vi "SeCrTs-RT_DAQ_- Copy.vi"(8 "error in":errorcluster, 9 "er":refnum<queue>, 11 "Data FIFO Ref":T1) -> (0 "error out":errorcluster)   [LabVIEW 2022 SP3]
uses:
  RT Controls/SeCrTs-Data FIFO.ctl
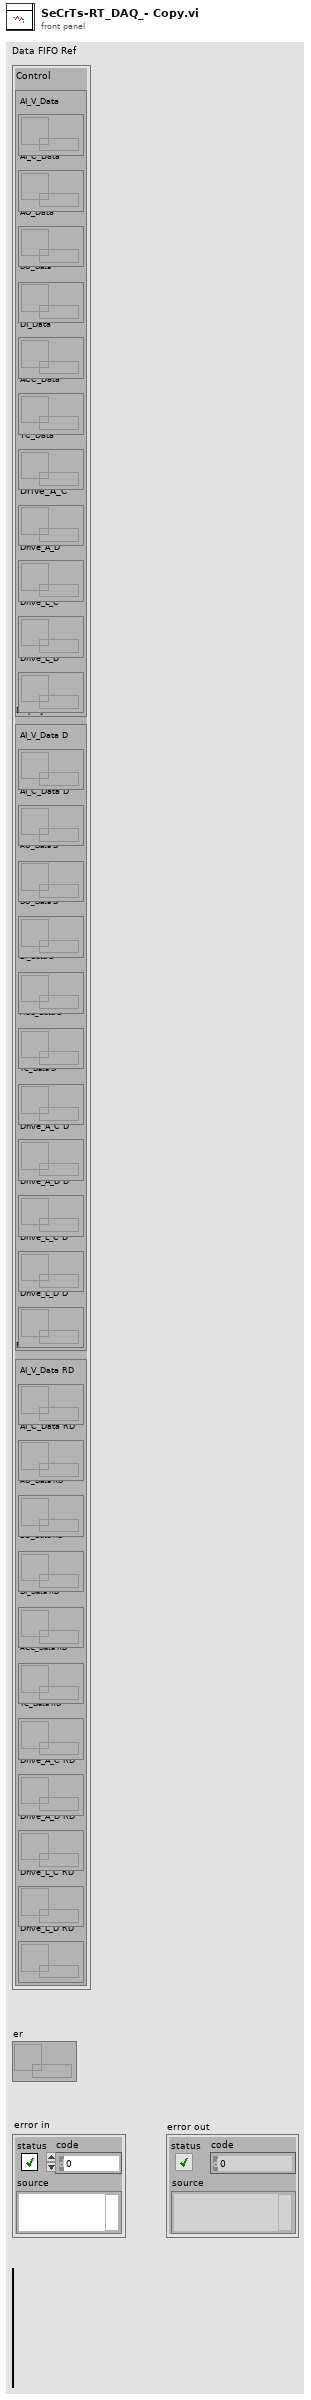
[diagram p1: front panel]
types:
  T1 = typedef "SeCrTs-Data FIFO.ctl" = cluster{"Control":cluster{"AI_V_Data":refnum<queue>, "AI_C_Data":refnum<queue>, "AO_Data":refnum<queue>, "DO_Data":refnum<queue>, "DI_Data":refnum<queue>, "ACC_Data":refnum<queue>, "TC_Data":refnum<queue>, "Drive_A_C":refnum<queue>, "Drive_A_D":refnum<queue>, "Drive_L_C":refnum<queue>, "Drive_L_D":refnum<queue>}, "Display":cluster{"AI_V_Data D":refnum<queue>, "AI_C_Data D":refnum<queue>, "AO_Data D":refnum<queue>, "DO_Data D":refnum<queue>, "DI_Data D":refnum<queue>, "ACC_Data D":refnum<queue>, "TC_Data D":refnum<queue>, "Drive_A_C D":refnum<queue>, "Drive_A_D D":refnum<queue>, "Drive_L_C D":refnum<queue>, "Drive_L_D D":refnum<queue>}, "RD":cluster{"AI_V_Data RD":refnum<queue>, "AI_C_Data RD":refnum<queue>, "AO_Data RD":refnum<queue>, "DO_Data RD":refnum<queue>, "DI_Data RD":refnum<queue>, "ACC_Data RD":refnum<queue>, "TC_Data RD":refnum<queue>, "Drive_A_C RD":refnum<queue>, "Drive_A_D RD":refnum<queue>, "Drive_L_C RD":refnum<queue>, "Drive_L_D RD":refnum<queue>}}
  T2 = cluster{"AO config":cluster{"Channel_Name":string, "Channel_Number":string, "Default_Value":dbl, "Units":string}[], "AI config":cluster{"Channel_Name":string, "Channel_Number":string, "Pre_Scale_min":dbl, "Pre_Scale_max":dbl, "Sensor_min":dbl, "Sensor_max":dbl, "Units":string}[], "DI config":cluster{"Channel_Name":string, "Channel_Number":string, "Default_Value":bool, "DI invert?":bool}[], "DO config":cluster{"Channel_Name":string, "Channel_Number":string, "Default_Value":bool, "DO invert?":bool}[], "TC config":cluster{"Channel_Name":string, "Channel_Number":string, "Pre_Scale_min":dbl, "Pre_Scale_max":dbl, "units":i32, " type":i32}[], "ACC config":cluster{"Channel_Name":string, "Channel_Number":string, "Pre_Scale_min":dbl, "Pre_Scale_max":dbl, "Terminal configuration":i32, "Sensitivity":dbl, "Sensitivity units":i32}[], "SG config":cluster{"Channel_Name":string, "Channel_Number":string, "Pre_Scale_min":dbl, "Pre_Scale_max":dbl}[], "Strain Gauge Settings":cluster{"poisson ratio":dbl, "nominal gage resistance":dbl, "gage factor":dbl}, "Bridge Settings":cluster{"voltage excitation value":dbl, "voltage excitation source":i32, "initial bridge voltage":dbl, "lead wire resistance":dbl, "strain configuration":i32}, "Sample Rate":cluster{"AI Sample Rate":dbl[], "AO Sample Rate":dbl[], "DI Sample Rate":dbl[], "TC Sample Rate":dbl[], "DO Sample Rate":dbl[], "SG Sample Rate":dbl[], "ACC Sample Rate":dbl[]}}
  T3 = enum16{"Initialize", "Create Task", "Start", "Acquire", "Stop", "Exit"}
  T4 = cluster{"AI_Task":refnum<k21>, "AO_Task":refnum<k21>, "DI_Task":refnum<k21>, "DO_Task":refnum<k21>, "ACC_Task":refnum<k21>, "TC_Task":refnum<k21>, "AI_V_Task":refnum<k21>}
  T5 = cluster{"Start DAQ":bool, "Stop DAQ":bool, "RT Stop":bool, "RT Exit":bool, "Start Seq":bool}
  T6 = cluster{"AO config":cluster{"Channel_Name":string, "Channel_Number":string, "Default_Value":dbl, "Units":string}[], "AI config":cluster{"Channel_Name":string, "Channel_Number":string, "Pre_Scale_min":dbl, "Pre_Scale_max":dbl, "Sensor_min":dbl, "Sensor_max":dbl, "Units":string}[], "DI config":cluster{"Channel_Name":string, "Channel_Number":string, "Default_Value":bool, "DI invert?":bool}[], "DO config":cluster{"Channel_Name":string, "Channel_Number":string, "Default_Value":bool, "DO invert?":bool}[], "TC config":cluster{"Channel_Name":string, "Channel_Number":string, "Pre_Scale_min":dbl, "Pre_Scale_max":dbl, "units":i32, "thermocouple type":i32}[], "ACC config":cluster{"Channel_Name":string, "Channel_Number":string, "Pre_Scale_min":dbl, "Pre_Scale_max":dbl, "Terminal configuration":i32, "Sensitivity":dbl, "Sensitivity units":i32}[], "SG config":cluster{"Channel_Name":string, "Channel_Number":string, "Pre_Scale_min":dbl, "Pre_Scale_max":dbl}[], "Strain Gauge Settings":cluster{"poisson ratio":dbl, "nominal gage resistance":dbl, "gage factor":dbl}, "Bridge Settings":cluster{"voltage excitation value":dbl, "voltage excitation source":i32, "initial bridge voltage":dbl, "lead wire resistance":dbl, "strain configuration":i32}, "Sample Rate":cluster{"AI Sample Rate":dbl[], "AO Sample Rate":dbl[], "DI Sample Rate":dbl[], "TC Sample Rate":dbl[], "DO Sample Rate":dbl[], "SG Sample Rate":dbl[], "ACC Sample Rate":dbl[]}}
  T7 = cluster{"Channel_Name":string, "Channel_Number":string, "Pre_Scale_min":dbl, "Pre_Scale_max":dbl, "Sensor_min":dbl, "Sensor_max":dbl, "Units":string}[]
  T8 = cluster{"Channel_Name":string, "Channel_Number":string, "Default_Value":dbl, "Units":string}[]
  T9 = cluster{"Channel_Name":string, "Channel_Number":string, "Default_Value":bool, "DI invert?":bool}[]
  T10 = cluster{"Channel_Name":string, "Channel_Number":string, "Default_Value":bool, "DO invert?":bool}[]
  T11 = cluster{"Channel_Name":string, "Channel_Number":string, "Pre_Scale_min":dbl, "Pre_Scale_max":dbl, "Terminal configuration":i32, "Sensitivity":dbl, "Sensitivity units":i32}[]
  T12 = cluster{"Channel_Name":string, "Channel_Number":string, "Pre_Scale_min":dbl, "Pre_Scale_max":dbl, "units":i32, " type":i32}[]
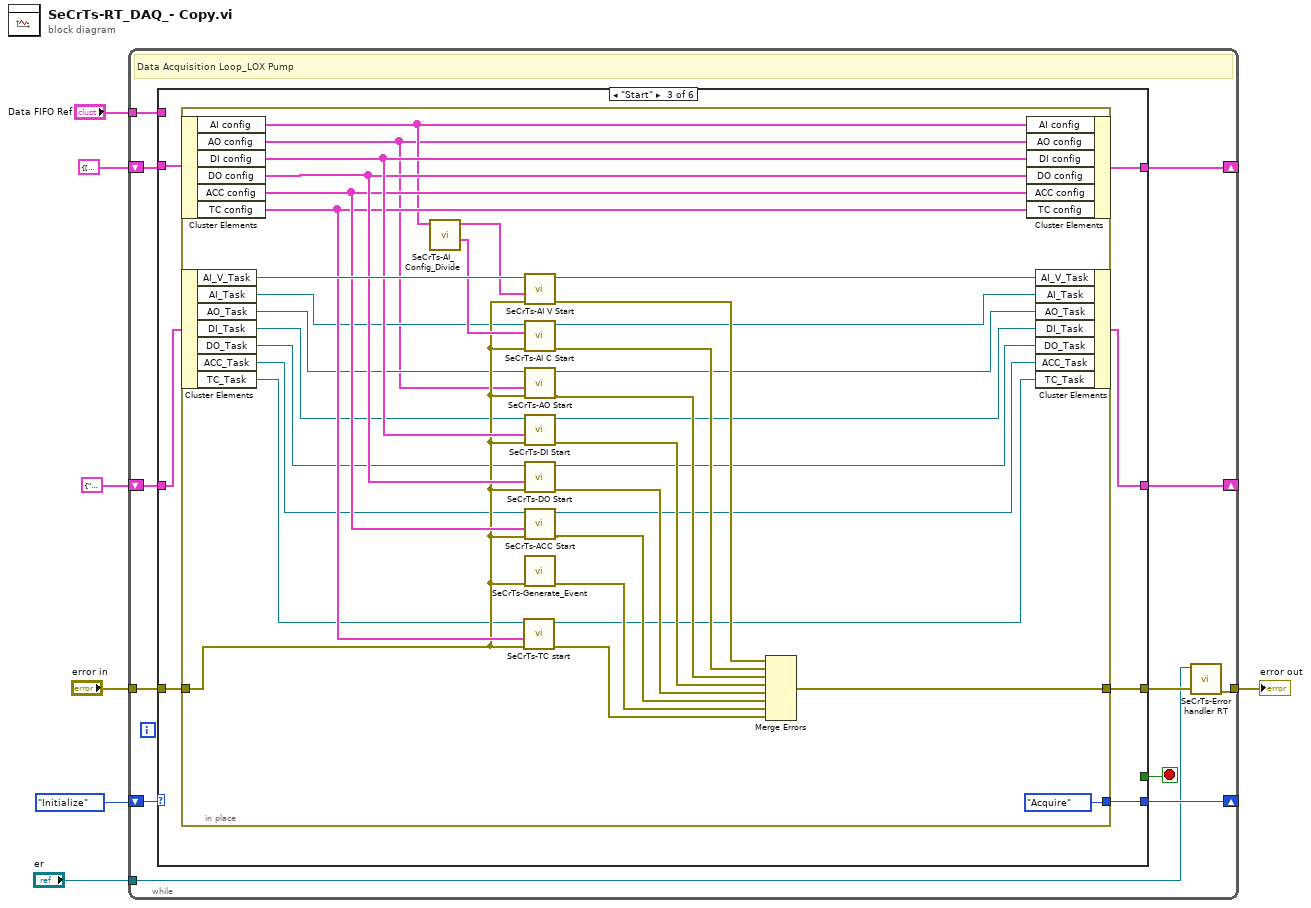
[diagram p0: block diagram]
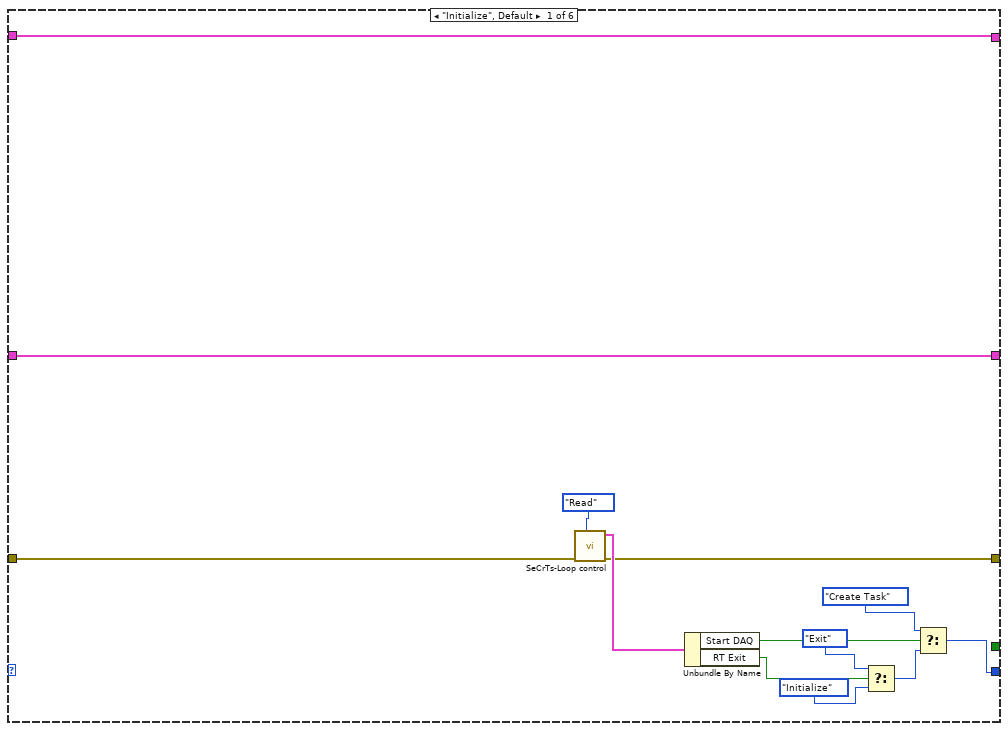
[diagram p2: hidden frame]
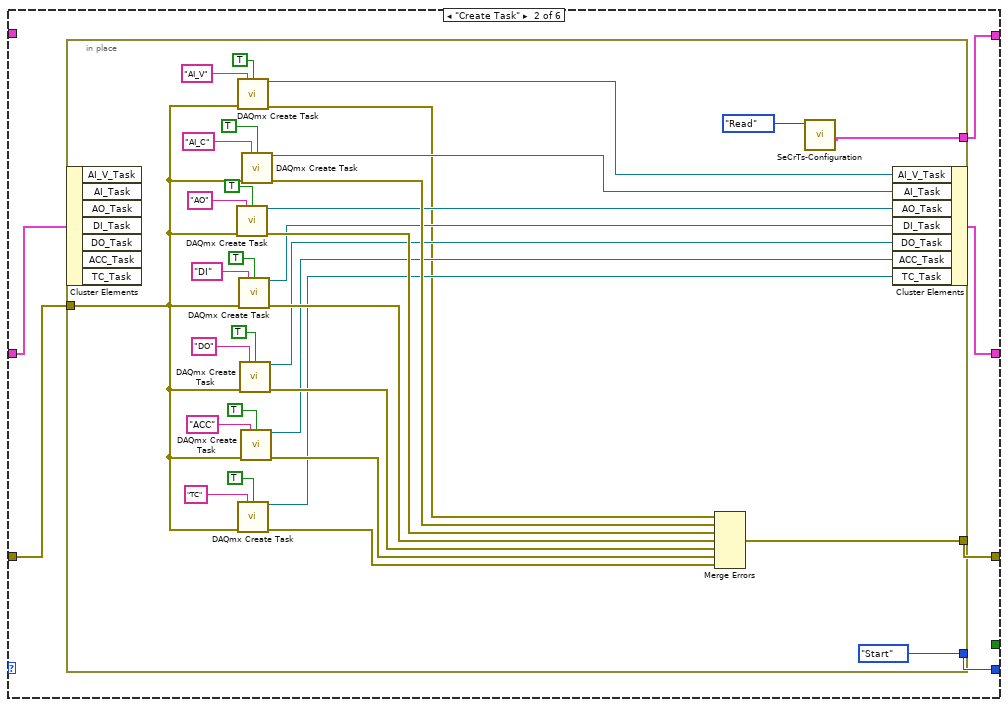
[diagram p3: hidden frame]
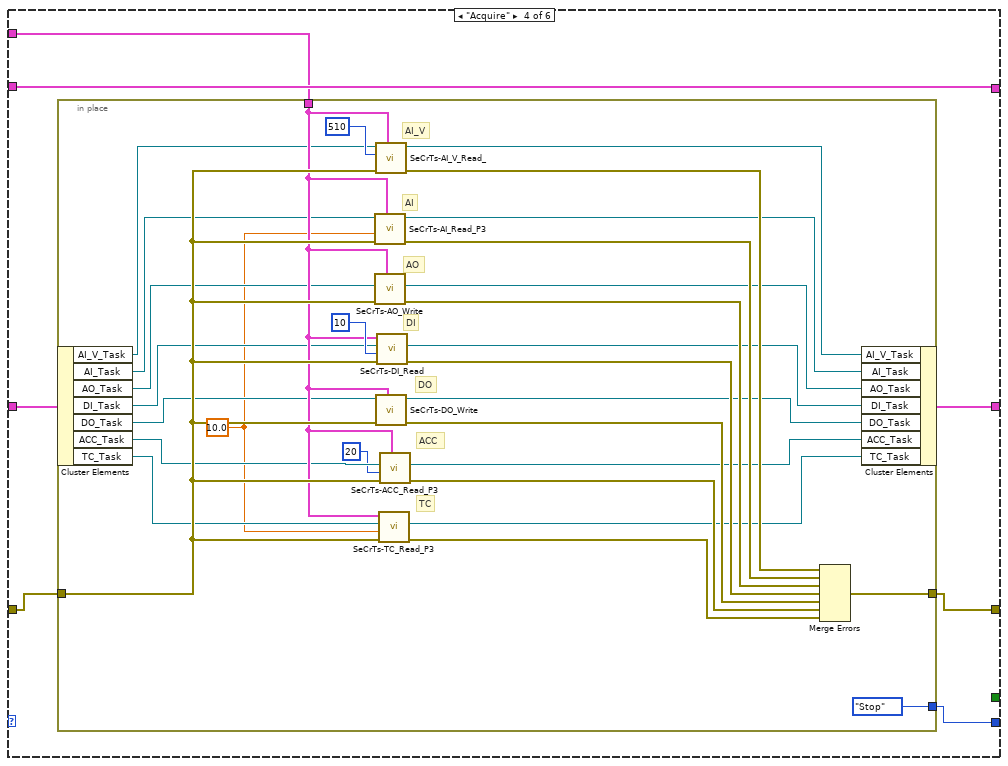
[diagram p4: hidden frame]
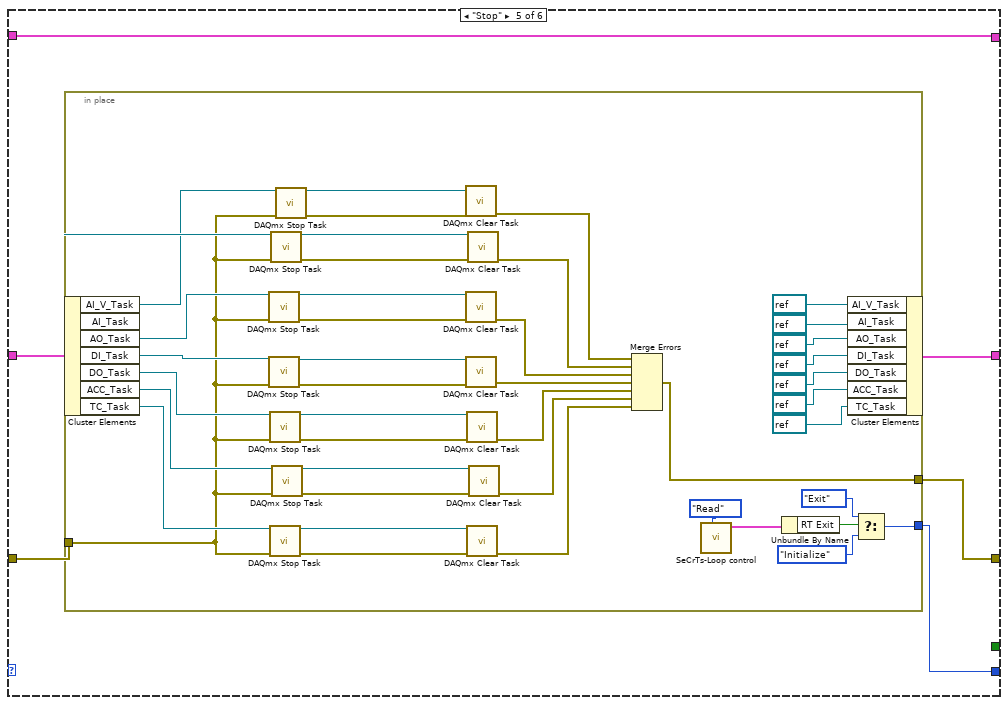
[diagram p5: hidden frame]
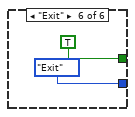
[diagram p6: hidden frame]
diagram:
  n1 = while {
    shift-right: [w17] -> _
    shift-left: T3."Initialize" -> [w19]
    tunnel: "error in" -> [w18]
    tunnel: [w8] -> w6
    shift-right: [w14] -> _
    shift-left: T2 {"AO config"=[], "AI config"=[], "DI config"=[], "DO config"=[], "TC config"=[], "ACC config"=[], "SG config"=[], "Strain Gauge Settings"={"poisson ratio"=0.0, "nominal gage resistance"=0.0, "gage factor"=0.0}, "Bridge Settings"={"voltage excitation value"=0.0, "voltage excitation source"=0, "initial bridge voltage"=0.0, "lead wire resistance"=0.0, "strain configuration"=0}, "Sample Rate"={"AI Sample Rate"=[], "AO Sample Rate"=[], "DI Sample Rate"=[], "TC Sample Rate"=[], "DO Sample Rate"=[], "SG Sample Rate"=[], "ACC Sample Rate"=[]}} ("Config out") -> [w15]
    shift-right: [w12] -> _
    shift-left: T4 {"AI_Task"="", "AO_Task"="", "DI_Task"="", "DO_Task"="", "ACC_Task"="", "TC_Task"="", "AI_V_Task"=""} -> [w16]
    tunnel: "Data FIFO Ref" -> [w11]
    tunnel: "er" -> [w9]
    stop <- w13 stop-if-true
    # "Data Acquisition Loop_LOX Pump"
    n2 = case shown="\"Start\"" w19 {
      tunnel: w18 -> [w21 w37 w77 w117 w151 _]
      tunnel: [w20 w36 w73 w116 w152 _] -> w10
      tunnel: [w31 w35 w78 w118 w153 T3."Exit"] -> w17
      tunnel: w16 -> [w23 w34 w76 w113 w150 _]
      tunnel: w15 -> [w22 _ w75 w115 w148 _]
      tunnel: [w22 w38 w74 w115 w148 _] -> w14
      tunnel: [_ _ _ _ _ TRUE] -> w13
      tunnel: [w23 w33 w72 w112 w149 _] -> w12
      tunnel: w11 -> [_ _ _ w114 _ _]
      frame "Initialize", Default {
        n3 = call "SeCrTs-Loop control.vi"("Action"=enum16{"Init", "Write", "Read"}."Read", "error in (no error)"=w21) -> ("error Out"=w20:errorcluster, "Loop Control out"=w27:T5)  [unwired: 8 in]
        n4 = Unbundle By Name(w27) -> ("Start DAQ"=w26:bool, "RT Exit"=w25:bool)
        n5 = Select(t=T3."Exit", s=w25, f=T3."Initialize") -> (s? t:f=w28:T3)
        n6 = Select(t=T3."Create Task", s=w26, f=w28) -> (s? t:f=w31:T3)
      }
      frame "Create Task" {
        n7 = in-place "In Place Element Structure" {
          in-place-border: [w50] -> w38
          in-place-border: w37 -> [w39]
          in-place-border: [w60] -> w36
          in-place-border: [T3."Start"] -> w35
          n8 = in-place-cluster #1(w34) -> ()  [unwired: 7 out]
          n9 = call <vilib>:"DAQmx Create Task.vi"("new task name"="AO", "auto cleanup"=TRUE, "error in"=w39) -> ("task out"=w58:refnum<k21>, "error out"=w65:errorcluster)  [unwired: 11 in]
          n10 = call <vilib>:"DAQmx Create Task.vi"("new task name"="AI_V", "auto cleanup"=TRUE, "error in"=w39) -> ("task out"=w51:refnum<k21>, "error out"=w40:errorcluster)  [unwired: 11 in]
          n11 = call <vilib>:"DAQmx Create Task.vi"("new task name"="TC", "auto cleanup"=TRUE, "error in"=w39) -> ("task out"=w54:refnum<k21>, "error out"=w61:errorcluster)  [unwired: 11 in]
          n12 = call <vilib>:"DAQmx Create Task.vi"("new task name"="DI", "auto cleanup"=TRUE, "error in"=w39) -> ("task out"=w57:refnum<k21>, "error out"=w64:errorcluster)  [unwired: 11 in]
          n13 = call <vilib>:"DAQmx Create Task.vi"("new task name"="DO", "auto cleanup"=TRUE, "error in"=w39) -> ("task out"=w56:refnum<k21>, "error out"=w63:errorcluster)  [unwired: 11 in]
          n14 = call <vilib>:"DAQmx Create Task.vi"("new task name"="ACC", "auto cleanup"=TRUE, "error in"=w39) -> ("task out"=w55:refnum<k21>, "error out"=w62:errorcluster)  [unwired: 11 in]
          n15 = call <vilib>:"DAQmx Create Task.vi"("new task name"="AI_C", "auto cleanup"=TRUE, "error in"=w39) -> ("task out"=w59:refnum<k21>, "error out"=w71:errorcluster)  [unwired: 11 in]
          n16 = Merge Errors(w40, w71, w65, w64, w63, w62, w61) -> (w60:errorcluster)
          n17 = call "SeCrTs-Configuration.vi"("Enum"=enum16{"Write", "Read"}."Read") -> ("Config out"=w50:T6)  [unwired: 10 in]
          n18 = in-place-cluster #1("AI_V_Task"=w51, "AI_Task"=w59, "AO_Task"=w58, "DI_Task"=w57, "DO_Task"=w56, "ACC_Task"=w55, "TC_Task"=w54) -> (w33:T4)
        }
      }
      frame "Start" {
        n19 = in-place "In Place Element Structure" {
          in-place-border: [T3."Acquire"] -> w78
          in-place-border: w77 -> [w97]
          in-place-border: [w92] -> w73
          n20 = in-place-cluster #2(w75) -> ("AI config"=w104:T7, "AO config"=w79:T8, "DI config"=w108:T9, "DO config"=w107:T10, "ACC config"=w106:T11, "TC config"=w105:T12)
          n21 = in-place-cluster #3(w76) -> ("AI_V_Task"=w110:refnum<k21>, "AI_Task"=w91:refnum<k21>, "AO_Task"=w90:refnum<k21>, "DI_Task"=w89:refnum<k21>, "DO_Task"=w88:refnum<k21>, "ACC_Task"=w87:refnum<k21>, "TC_Task"=w86:refnum<k21>)
          n22 = call "SeCrTs-AI_Config_Divide.vi"("AI config"=w104) -> ("AI C"=w102:T7, "AI V"=w103:T7)  [unwired: 9 in]
          n23 = call "SeCrTs-TC start .vi"("error in"=w97, "TC config"=w105, "Refnum in"=w86) -> ("error out"=w93:errorcluster, "Refnum out"=w80:refnum<k21>)  [unwired: 7 in]
          n24 = call "SeCrTs-AI V Start .vi"("error in"=w97, "AI V"=w103, "Refnum in"=w110) -> ("error out"=w101:errorcluster, "Refnum out"=w109:refnum<k21>)  [unwired: 7 in]
          n25 = call "SeCrTs-AI C Start .vi"("error in"=w97, "AI C"=w102, "Refnum in"=w91) -> ("error out"=w100:errorcluster, "Refnum out"=w85:refnum<k21>)  [unwired: 7 in]
          n26 = call "SeCrTs-AO Start .vi"("error in"=w97, "AO config"=w79, "Refnum in"=w90) -> ("error out"=w99:errorcluster, "Refnum out"=w84:refnum<k21>)  [unwired: 7 in]
          n27 = call "SeCrTs-DI Start.vi"("error in"=w97, "DI config"=w108, "Refnum in"=w89) -> ("error out"=w98:errorcluster, "Refnum out"=w83:refnum<k21>)  [unwired: 7 in]
          n28 = call "SeCrTs-DO Start.vi"("error in"=w97, "DO config"=w107, "Refnum in"=w88) -> ("error out"=w96:errorcluster, "Refnum out"=w82:refnum<k21>)  [unwired: 7 in]
          n29 = call "SeCrTs-ACC Start.vi"("error in"=w97, "ACC config"=w106, "Refnum in"=w87) -> ("error out"=w95:errorcluster, "Refnum out"=w81:refnum<k21>)  [unwired: 7 in]
          n30 = call "SeCrTs-Generate_Event.vi"("error in"=w97) -> ("error out"=w94:errorcluster)  [unwired: 10 in]
          n31 = Merge Errors(w101, w100, w99, w98, w96, w95, w94, w93) -> (w92:errorcluster)
          n32 = in-place-cluster #2("AI config"=w104, "AO config"=w79, "DI config"=w108, "DO config"=w107, "ACC config"=w106, "TC config"=w105) -> (w74:T2)
          n33 = in-place-cluster #3("AI_V_Task"=w109, "AI_Task"=w85, "AO_Task"=w84, "DI_Task"=w83, "DO_Task"=w82, "ACC_Task"=w81, "TC_Task"=w80) -> (w72:T4)
        }
      }
      frame "Acquire" {
        n34 = in-place "In Place Element Structure" {
          in-place-border: [T3."Stop"] -> w118
          in-place-border: w117 -> [w138]
          in-place-border: [w146] -> w116
          in-place-border: w114 -> [w136]
          w120 = 10.0
          # "AO"
          # "ACC"
          # "AI_V"
          # "TC"
          # "DO"
          # "DI"
          # "AI"
          n35 = in-place-cluster #4(w113) -> ("AI_V_Task"=w121:refnum<k21>, "AI_Task"=w135:refnum<k21>, "AO_Task"=w134:refnum<k21>, "DI_Task"=w133:refnum<k21>, "DO_Task"=w132:refnum<k21>, "ACC_Task"=w131:refnum<k21>, "TC_Task"=w130:refnum<k21>)
          n36 = call "SeCrTs-AI_Read_P3.vi"("Data FIFO Ref"=w136, "error in (no error)"=w138, "Numeric"=w120, "AI_Task"=w135) -> ("error out"=w144:errorcluster, "task out"=w128:refnum<k21>)  [unwired: 4 in]
          n37 = call "SeCrTs-AO_Write.vi"("Data FIFO Ref"=w136, "error in (no error)"=w138, "AO_Task"=w134) -> ("error out"=w143:errorcluster, "task out"=w127:refnum<k21>)  [unwired: 7 in]
          n38 = call "SeCrTs-AI_V_Read_.vi"("Data FIFO Ref"=w136, "error in"=w138, "number of samples per channel"=510, "AI_V_Task"=w121) -> ("error out"=w145:errorcluster, "AI_V_Task"=w129:refnum<k21>)  [unwired: 6 in]
          n39 = call "SeCrTs-DO_Write.vi"("Data FIFO Ref"=w136, "error in (no error)"=w138, "Refnum in"=w132) -> ("error out"=w141:errorcluster, "Refnum out"=w125:refnum<k21>)  [unwired: 7 in]
          n40 = call "SeCrTs-DI_Read.vi"("error in (no error)"=w138, "number of samples per channel"=10, "DI_Task"=w133, "Data FIFO Ref"=w136) -> ("error out"=w142:errorcluster, "task out"=w126:refnum<k21>)  [unwired: 6 in]
          n41 = call "SeCrTs-TC_Read_P3.vi"("error in (no error)"=w138, "Numeric"=w120, "TC_Task"=w130, "Data FIFO Ref"=w136) -> ("error out"=w139:errorcluster, "task out"=w123:refnum<k21>)  [unwired: 6 in]
          n42 = call "SeCrTs-ACC_Read_P3.vi"("Data FIFO Ref"=w136, "error in (no error)"=w138, "number of samples per channel"=20, "ACC_Task"=w131) -> ("error out"=w140:errorcluster, "task out"=w124:refnum<k21>)  [unwired: 6 in]
          n43 = Merge Errors(w145, w144, w143, w142, w141, w140, w139) -> (w146:errorcluster)
          n44 = in-place-cluster #4("AI_V_Task"=w129, "AI_Task"=w128, "AO_Task"=w127, "DI_Task"=w126, "DO_Task"=w125, "ACC_Task"=w124, "TC_Task"=w123) -> (w112:T4)
        }
      }
      frame "Stop" {
        n45 = in-place "In Place Element Structure" {
          in-place-border: [w193] -> w153
          in-place-border: [w187] -> w152
          in-place-border: w151 -> [w168]
          n46 = in-place-cluster #5(w150) -> ("AI_V_Task"=w170:refnum<k21>, "AI_Task"=w179:refnum<k21>, "AO_Task"=w178:refnum<k21>, "DI_Task"=w181:refnum<k21>, "DO_Task"=w180:refnum<k21>, "ACC_Task"=w177:refnum<k21>, "TC_Task"=w176:refnum<k21>)
          n47 = call <vilib>:"DAQmx Stop Task.vi"("task/channels in"=w178, "error in"=w168) -> ("task out"=w175:refnum<k21>, "error out"=w192:errorcluster)  [unwired: 12 in]
          n48 = call <vilib>:"DAQmx Stop Task.vi"("task/channels in"=w181, "error in"=w168) -> ("task out"=w174:refnum<k21>, "error out"=w191:errorcluster)  [unwired: 12 in]
          n49 = call <vilib>:"DAQmx Stop Task.vi"("task/channels in"=w180, "error in"=w168) -> ("task out"=w173:refnum<k21>, "error out"=w190:errorcluster)  [unwired: 12 in]
          n50 = call <vilib>:"DAQmx Stop Task.vi"("task/channels in"=w176, "error in"=w168) -> ("task out"=w171:refnum<k21>, "error out"=w188:errorcluster)  [unwired: 12 in]
          n51 = call <vilib>:"DAQmx Stop Task.vi"("task/channels in"=w179, "error in"=w168) -> ("task out"=w156:refnum<k21>, "error out"=w155:errorcluster)  [unwired: 12 in]
          n52 = call <vilib>:"DAQmx Stop Task.vi"("task/channels in"=w177, "error in"=w168) -> ("task out"=w172:refnum<k21>, "error out"=w189:errorcluster)  [unwired: 12 in]
          n53 = call <vilib>:"DAQmx Stop Task.vi"("task/channels in"=w170, "error in"=w168) -> ("task out"=w169:refnum<k21>, "error out"=w167:errorcluster)  [unwired: 12 in]
          n54 = call <vilib>:"DAQmx Clear Task.vi"("task in"=w169, "error in"=w167) -> ("error out"=w166:errorcluster)  [unwired: 13 in]
          n55 = call <vilib>:"DAQmx Clear Task.vi"("task in"=w175, "error in"=w192) -> ("error out"=w186:errorcluster)  [unwired: 13 in]
          n56 = call <vilib>:"DAQmx Clear Task.vi"("task in"=w174, "error in"=w191) -> ("error out"=w185:errorcluster)  [unwired: 13 in]
          n57 = call <vilib>:"DAQmx Clear Task.vi"("task in"=w173, "error in"=w190) -> ("error out"=w184:errorcluster)  [unwired: 13 in]
          n58 = call <vilib>:"DAQmx Clear Task.vi"("task in"=w171, "error in"=w188) -> ("error out"=w182:errorcluster)  [unwired: 13 in]
          n59 = call <vilib>:"DAQmx Clear Task.vi"("task in"=w156, "error in"=w155) -> ("error out"=w196:errorcluster)  [unwired: 13 in]
          n60 = call <vilib>:"DAQmx Clear Task.vi"("task in"=w172, "error in"=w189) -> ("error out"=w183:errorcluster)  [unwired: 13 in]
          n61 = Merge Errors(w166, w196, w186, w185, w184, w183, w182) -> (w187:errorcluster)
          n62 = call "SeCrTs-Loop control.vi"("Action"=enum16{"Init", "Write", "Read"}."Read") -> ("Loop Control out"=w165:T5)  [unwired: 9 in, 1 out]
          n63 = Unbundle By Name(w165) -> ("RT Exit"=w164:bool)
          n64 = in-place-cluster #5("AI_V_Task"=refnum<k21> refnum, "AI_Task"=refnum<k21> refnum, "AO_Task"=refnum<k21> refnum, "DI_Task"=refnum<k21> refnum, "DO_Task"=refnum<k21> refnum, "ACC_Task"=refnum<k21> refnum, "TC_Task"=refnum<k21> refnum) -> (w149:T4)
          n65 = Select(t=T3."Exit", s=w164, f=T3."Initialize") -> (s? t:f=w193:T3)
        }
      }
      frame "Exit" {
      }
    }
    n66 = call "SeCrTs-Error handler RT.vi"("error in"=w10, "Message Queue"=w9) -> ("error out"=w8:errorcluster)  [unwired: 8 in, 1 out]
  }
  "error out" <- w6
